vi "Close.vi"(8 "error in (no error)":errorcluster, 11 "Abstract UUT in":refnum<class "Abstract UUT.lvclass">) -> (0 "error out":errorcluster, 3 "Abstract UUT out":refnum<class "Abstract UUT.lvclass">)   [LabVIEW 2019, in "Sequence Main.lvlib" / "Abstract UUT.lvclass"]
uses:
  Abstract UUT.lvclass
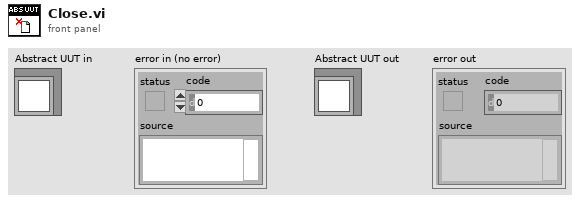
[diagram p1: front panel]
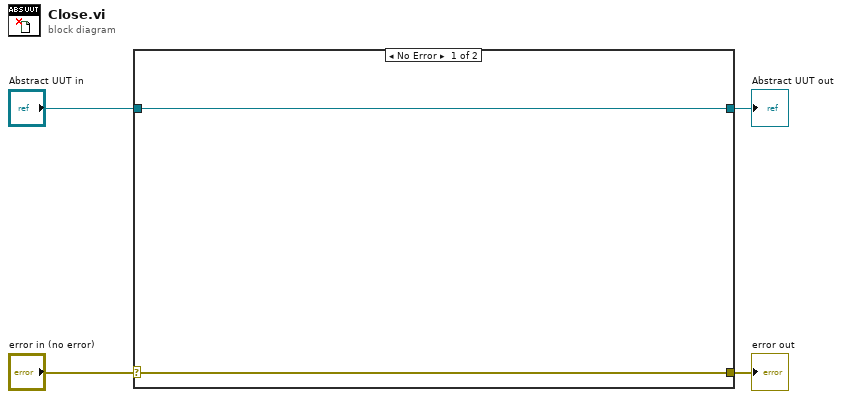
[diagram p0: block diagram]
diagram:
  n1 = case shown="No Error" "error in (no error)" {
    selector: "error in (no error)" -> [w5 w8]
    tunnel: [w5 w8] -> w3
    tunnel: [w6 w7] -> w1
    tunnel: "Abstract UUT in" -> [w6 w7]
    frame No Error {
    }
    frame Error {
    }
  }
  "error out" <- w3
  "Abstract UUT out" <- w1
